vi "Expt9 niUSRP EX PSK Tx student.vi"() -> ()   [LabVIEW 2020]
doc: "This example <B>requires the Modulation Toolkit</B>.\n\nApplies PSK (Phase Shift Keyed Modulation) to a PN sequence for USRP-based transmission. Continuously transmits a repeating message with a length determined by the PN Sequence Order parameter. \n\nThis example is paired with the example \"niUSRP Ex PSK Rx.vi\", which allows you to establish a Tx / Rx link between two separate USRPs. \n\nTo establish a Tx / Rx link between two USRPs:\n1) Ensure that the Tx and Rx example VIs have matching parameters for Modulation Scheme (M-Ary), Carrier Frequency, and Symbol Rate. Specify the Symbol Rate by setting the combination of the IQ Sampling Rate and the Number of Samples per Symbol parameters.\n2) Choose an IQ Sample Rate that enables sufficient Rx bandwidth.\n3) Set the Tx and / or Rx gain to ensure a sufficient signal to noise ratio on the Receive side. Note: applying too much gain can result in clipping.\n4) Choose a sufficient acquisition frame length to enable the demodulator to lock to the transmitted signal. National Instruments recommends that the acquired frame contain a number of symbols that is at least 20 * M-Ary of the modulation scheme. \n5) Ensure that the Reset Demodulator control is set to True until a solid lock is established. \n6) Install antennas and attenuators that efficiently operate at the carrier frequency you choose."
uses:
  <instrlib>/niUSRP/niUSRP Write Tx Data (CDB Cluster).vi
  <vilib>/addons/Modulation/niDMT.lvlib
panel:
  out "error out":errorcluster
  in  "Enabled Channel":string(combo)="0"
  out "Gain [dB] (actual)":dbl=12.0 format="%#.6p"
  out "Carrier Frequency \n[Hz] (actual)":dbl=915000000.0 format="%#.6p"
  out "IQ Sampling\nRate [S/sec] (actual)":dbl=500000.0 format="%#.6p"
  in  "Active Antenna":string(combo)="TX1"
  in  "Gain [dB]":dbl=12.0 format="%#.6p"
  in  "Carrier\nFrequency [Hz]":dbl=915000000.0 format="%#.6p"
  in  "IQ Sampling\nRate [S/sec]":dbl=500000.0 format="%#.6p"
  in  "Device Name":refnum<k15>="192.168.10.5"
  in  "Choose a PSK Format":T1(tab)=enum."8-PSK" caption="PSK"
  in  "BPSK System Parameters":T2={"Samples per Symbol"=8, "symbol map"=[], "Differential PSK"=enum."disable", "PSK type"=0} {"PSK type" items=["normal", "shifted", "offset"]; "symbol map" format="%.3f"}
  in  "QPSK System Parameters":T2={"Samples per Symbol"=8, "symbol map"=[], "Differential PSK"=enum."disable", "PSK type"=0} {"PSK type" items=["normal", "shifted", "offset"]; "symbol map" format="%.3f"}
  in  "pi/4 DQPSK System Parameters":T2={"Samples per Symbol"=8, "symbol map"=[], "Differential PSK"=enum."enable", "PSK type"=1} {"PSK type" items=["normal", "shifted", "offset"]; "symbol map" format="%.3f"}
  in  "OQPSK System Parameters":T2={"Samples per Symbol"=8, "symbol map"=[], "Differential PSK"=enum."disable", "PSK type"=2} {"PSK type" items=["normal", "shifted", "offset"]; "symbol map" format="%.3f"}
  in  "8-PSK System Parameters":T2={"Samples per Symbol"=4, "symbol map"=[], "Differential PSK"=enum."disable", "PSK type"=0} {"PSK type" items=["normal", "shifted", "offset"]; "symbol map" format="%.3f"}
  in  "16-PSK System Parameters":T2={"Samples per Symbol"=8, "symbol map"=[], "Differential PSK"=enum."disable", "PSK type"=0} {"PSK type" items=["normal", "shifted", "offset"]; "symbol map" format="%.3f"}
  in  "M":i32=4 min=2 step=2
  in  "Custom System Parameters":T2={"Samples per Symbol"=8, "symbol map"=[], "Differential PSK"=enum."disable", "PSK type"=0} {"PSK type" items=["normal", "shifted", "offset"]; "symbol map" format="%.3f"}
  out "Frame Size [samples]":i32=4092
  in  "Pn Sequence Order":i32=13
  in  "Filter Parameters":T3={"Alpha"=0.5, "Filter Length"=6, "TX Filter"=enum."Root Raised Cos"} {"Alpha" format="%.2f"}
  out "Symbol Rate\n[symbols/sec]":dbl=500000.0 format="%#.6p"
  in  "Stop":bool
  out "Constellation Graph":T4(graph) caption="Tx Signal Constellation"
  # "Note:\nFrame size (samples per write) =\n (2^Pn Sequence Order) * Samples Per Symbol.\nUse Pn Sequence Order of 12 when using a 1 Gb Ethernet connection on a USRP RIO device. This prevents underflows by implicitly choosing \na frame size close to the ideal frame size for Ethernet connection. Refer to the \"Data Streaming Performance Tips\" section in the NI-USRP Help at ni.com/manuals for more information."
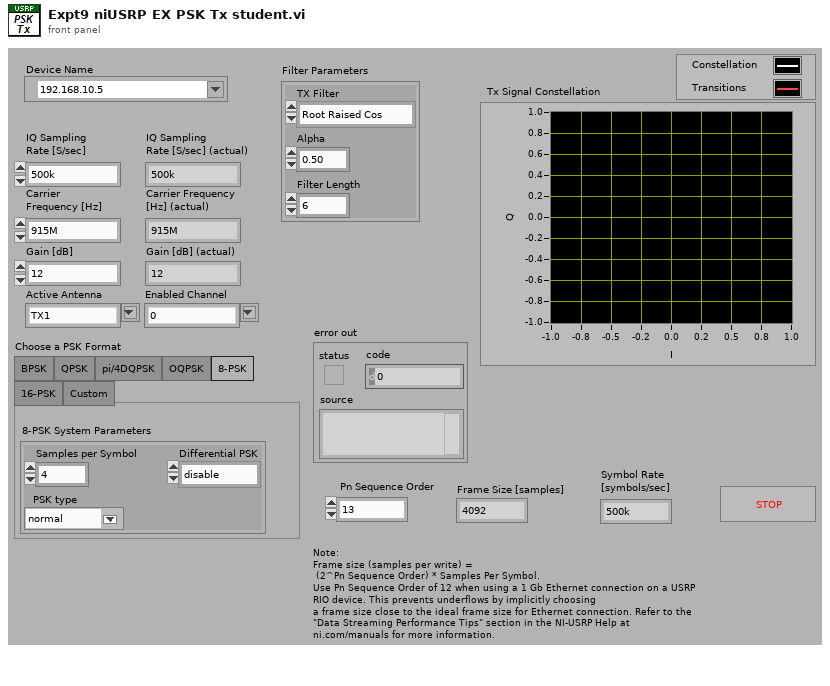
[diagram p1: front panel]
types:
  T1 = enum32{"BPSK", "QPSK", "pi/4DQPSK", "OQPSK", "8-PSK", "16-PSK", "Custom"}
  T2 = cluster{"Samples per Symbol":i32, "symbol map":cdb[], "Differential PSK":enum16{"disable", "enable"}, "PSK type":u16}
  T3 = cluster{"Alpha":dbl, "Filter Length":i32, "TX Filter":enum16{"none", "Raised Cosine", "Root Raised Cos", "Gaussian"}}
  T4 = cluster{"constellation":dbl[], "oversampled data":dbl[]}[]
  T5 = enum32{"PN sequence", "user-defined pattern", "Read from file"}
  T6 = typedef "niAMT.lvlib/Complex Data Waveform.ctl" = cluster{"t0":dbl, "dt":dbl, "Y":cdb[]}
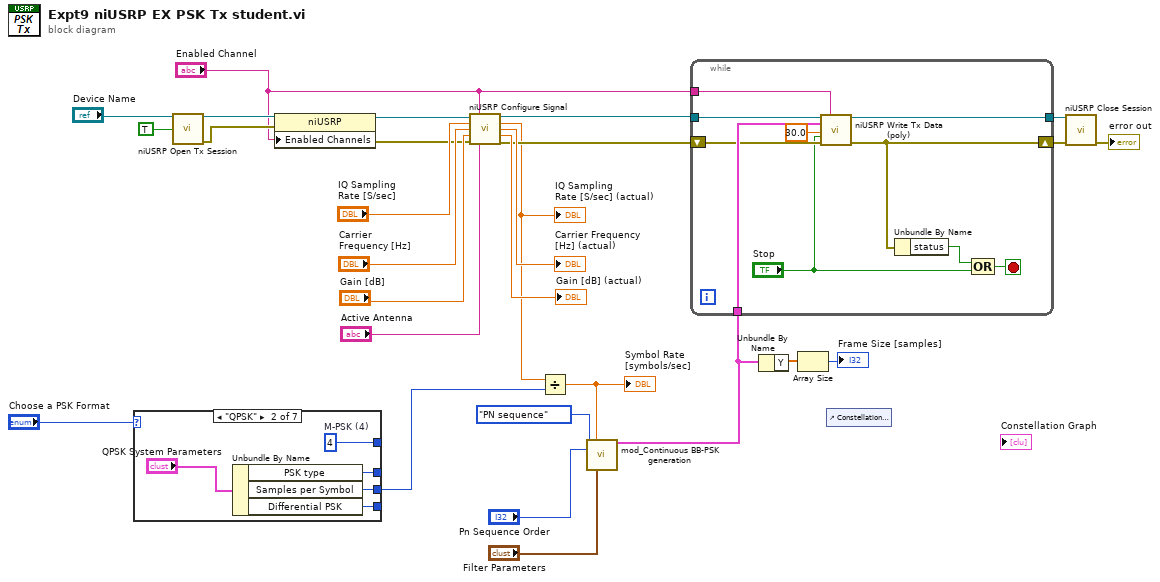
[diagram p0: block diagram]
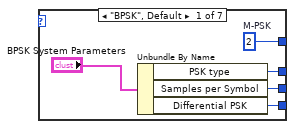
[diagram p2: hidden frame]
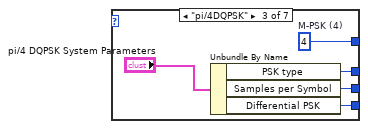
[diagram p3: hidden frame]
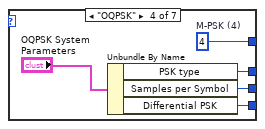
[diagram p4: hidden frame]
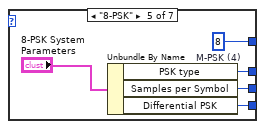
[diagram p5: hidden frame]
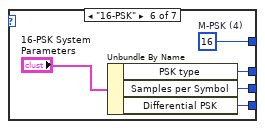
[diagram p6: hidden frame]
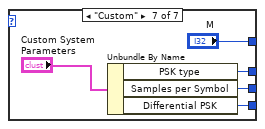
[diagram p7: hidden frame]
diagram:
  n1 = case shown="\"QPSK\"" "Choose a PSK Format" {
    tunnel: [w30 w37 w42 w47 w52 w58 w61] -> w7
    tunnel: [w31 w35 w41 w46 w51 w57 w62] -> _
    tunnel: [w33 w38 w43 w48 w50 w56 "M"] -> _
    tunnel: [w32 w36 w40 w45 w53 w55 w63] -> _
    frame "BPSK", Default {
      w33 = 2  # M-PSK
      n2 = Unbundle By Name("BPSK System Parameters") -> ("PSK type"=w32:u16, "Samples per Symbol"=w30:i32, "Differential PSK"=w31:enum16{"disable", "enable"})
    }
    frame "QPSK" {
      w38 = 4  # M-PSK (4)
      n3 = Unbundle By Name("QPSK System Parameters") -> ("PSK type"=w36:u16, "Samples per Symbol"=w37:i32, "Differential PSK"=w35:enum16{"disable", "enable"})
    }
    frame "pi/4DQPSK" {
      w43 = 4  # M-PSK (4)
      n4 = Unbundle By Name("pi/4 DQPSK System Parameters") -> ("PSK type"=w40:u16, "Samples per Symbol"=w42:i32, "Differential PSK"=w41:enum16{"disable", "enable"})
    }
    frame "OQPSK" {
      w48 = 4  # M-PSK (4)
      n5 = Unbundle By Name("OQPSK System Parameters") -> ("PSK type"=w45:u16, "Samples per Symbol"=w47:i32, "Differential PSK"=w46:enum16{"disable", "enable"})
    }
    frame "8-PSK" {
      w50 = 8  # M-PSK (4)
      n6 = Unbundle By Name("8-PSK System Parameters") -> ("PSK type"=w53:u16, "Samples per Symbol"=w52:i32, "Differential PSK"=w51:enum16{"disable", "enable"})
    }
    frame "16-PSK" {
      w56 = 16  # M-PSK (4)
      n7 = Unbundle By Name("16-PSK System Parameters") -> ("PSK type"=w55:u16, "Samples per Symbol"=w58:i32, "Differential PSK"=w57:enum16{"disable", "enable"})
    }
    frame "Custom" {
      n8 = Unbundle By Name("Custom System Parameters") -> ("PSK type"=w63:u16, "Samples per Symbol"=w61:i32, "Differential PSK"=w62:enum16{"disable", "enable"})
    }
  }
  n9 = call <instrlib>:"niUSRP Open Tx Session.vi"("device names"="Device Name", "reset"=TRUE) -> ("session handle out"=w6:refnum<k15>, "error out"=w5:errorcluster)  [unwired: 12 in]
  n10 = property class="niUSRP"(reference=w6, error in=w5, "Enabled Channels"="Enabled Channel") -> (reference out=w4:refnum<k15>, error out=w3:errorcluster)
  n11 = call <instrlib>:"niUSRP Configure Signal.vi"("session handle"=w4, "channel list"="Enabled Channel", "IQ rate"="IQ Sampling\nRate [S/sec]", "carrier frequency"="Carrier\nFrequency [Hz]", "gain"="Gain [dB]", "error in (no error)"=w3, "active antenna"="Active Antenna") -> ("session handle out"=w10:refnum<k15>, "coerced IQ rate"=w8:dbl, "coerced carrier frequency"=→"Carrier Frequency \n[Hz] (actual)":dbl, "coerced gain"=→"Gain [dB] (actual)":dbl, "error out"=w9:errorcluster)  [unwired: 4 in]
  "IQ Sampling\nRate [S/sec] (actual)" <- w8
  n12 = Divide(x=w8, y=w7) -> (x/y=w22:dbl)
  "Symbol Rate\n[symbols/sec]" <- w22
  n13 = call <vilib>:"mod_Continuous BB-PSK generation.vi"("bit stream type"=T5."PN sequence", "Symbol Rate, Hz"=w22, "PN Sequence Order"="Pn Sequence Order", "filter parameters"="Filter Parameters") -> ("output complex waveform"=w21:T6)  [unwired: 9 in, 2 out]
  n14 = while {
    tunnel: [w70] -> w19
    tunnel: w10 -> [w73]
    shift-right: [w66] -> w20
    shift-left: w9 -> [w71]
    tunnel: w21 -> [w72]
    tunnel: "Enabled Channel" -> [w65]
    stop <- w69 stop-if-true
    n15 = call-poly <instrlib>:"niUSRP Write Tx Data (poly).vi"("session handle"=w73, "channel list"=w65, "data"=w72, "timeout"=30.0, "end of data?"="Stop", "error in (no error)"=w71) -> ("session handle out"=w70:refnum<k15>, "error out"=w66:errorcluster)  [unwired: 8 in]
    n16 = Unbundle By Name(w66) -> ("status"=w68:bool)
    n17 = Compound Arithmetic op=OR(w68, "Stop") -> (w69:bool)
  }
  n18 = Unbundle By Name(w21) -> ("Y"=w28:cdb[])
  n19 = Array Size(array=w28) -> (size(s)=→"Frame Size [samples]":i32)
  n20 = control-ref of="Constellation Graph"() -> ()  [unwired: 1 out]
  n21 = call <instrlib>:"niUSRP Close Session.vi"("session handle"=w19, "error in (no error)"=w20) -> ("error out"=→"error out":errorcluster)  [unwired: 13 in]
